vi "decimal_to_string_array.vi"(9 "No. of display digits":i32=5, 11 "number in":dbl format="%#.10f") -> (0 "out of range?":bool, 1 "dot position":bool[](array[boolean]), 2 "number array":u16[](array[numeric]), 3 "negative?":bool)   [LabVIEW 2015]
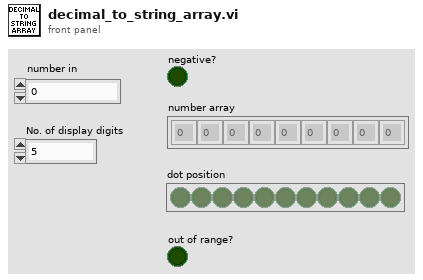
[diagram p1: front panel]
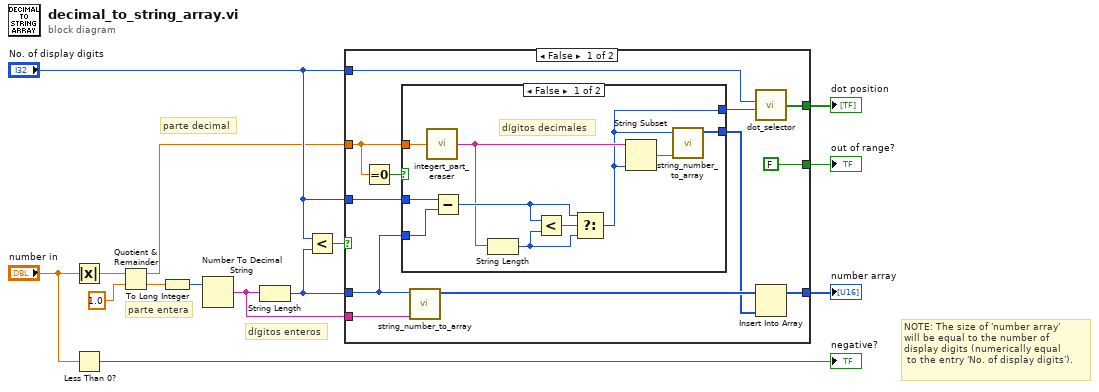
[diagram p0: block diagram]
diagram:
  # "NOTE: The size of 'number array'\nwill be equal to the number of \ndisplay digits (numerically equal\n to the entry 'No. of display digits')."
  # "dígitos enteros"
  # "parte decimal"
  # "parte entera"
  n1 = Absolute Value(x="number in") -> (abs(x)=w14:dbl)
  n2 = Less Than 0?(x="number in") -> (x < 0?=→"negative?":bool)
  n3 = Quotient & Remainder(x=w14, y=1.0) -> (x-y*floor(x/y)=w1:dbl, floor(x/y)=w11:dbl)
  n4 = To Long Integer(number=w11) -> (32bit integer=w12:i32)
  n5 = Number To Decimal String(number=w12) -> (decimal integer string=w9:string)  [unwired: 1 in]
  n6 = String Length(string=w9) -> (length=w4:i32)
  n7 = Less?(x="No. of display digits", y=w4) -> (x < y?=w5:bool)
  n8 = case shown="False" w5 {
    selector: w5 -> [_ w37]
    tunnel: w1 -> [w25 _]
    tunnel: [w22 _] -> w10
    tunnel: w9 -> [w15 _]
    tunnel: "No. of display digits" -> [w21 _]
    tunnel: w4 -> [w20 _]
    tunnel: [FALSE w37] -> w8
    tunnel: "No. of display digits" -> [w17 _]
    tunnel: [w16 _] -> w2
    frame False {
      n9 = Equal To 0?(x=w25) -> (x = 0?=w26:bool)
      n10 = case shown="False" w26 {
        tunnel: w20 -> [w36 _]
        tunnel: w25 -> [w29 _]
        tunnel: [w27 _] -> w18
        tunnel: [w30 _] -> w23
        tunnel: w21 -> [w32 _]
        frame False {
          # "dígitos decimales"
          n11 = call "integert_part_eraser.vi"("numeric"=w29) -> ("numeric string"=w28:string)  [unwired: 6 in]
          n12 = Subtract(x=w32, y=w36) -> (x-y=w33:i32)
          n13 = String Length(string=w28) -> (length=w34:i32)
          n14 = Less?(x=w33, y=w34) -> (x < y?=w35:bool)
          n15 = Select(t=w33, s=w35, f=w34) -> (s? t:f=w27:i32)
          n16 = String Subset(string=w28, length (rest)=w27) -> (substring=w31:string)  [unwired: 1 in]
          n17 = call "string_number_to_array.vi"("string number"=w31, "numeric length"=w27) -> ("array number"=w30:u16[])  [unwired: 9 in]
        }
        frame True {
        }
      }
      n18 = call "string_number_to_array.vi"("string number"=w15, "numeric length"=w20) -> ("array number"=w24:u16[])  [unwired: 9 in]
      n19 = call "dot_selector.vi"("n° digitos display"=w17, "decimal length"=w18) -> ("dot"=w16:bool[])  [unwired: 6 in]
      n20 = Insert Into Array(array=w24, new element=w23) -> (w22:u16[])  [unwired: 1 in]
    }
    frame True {
      # "Out of range"
    }
  }
  "number array" <- w10
  "out of range?" <- w8
  "dot position" <- w2
